vi "PWM_OUT.vi"() -> ()   [LabVIEW 2012]
uses:
  Usb_Daq_V52_Dll.dll
panel:
  in  "stop":bool
  in  "OK Button":bool
  in  "停止/运行":i32 min=0 max=1
  in  "占空比":sgl=1.0 min=1 max=99
  in  "频率":i32=1 min=1 max=100000
  in  "通道":i32=1 min=0 max=3
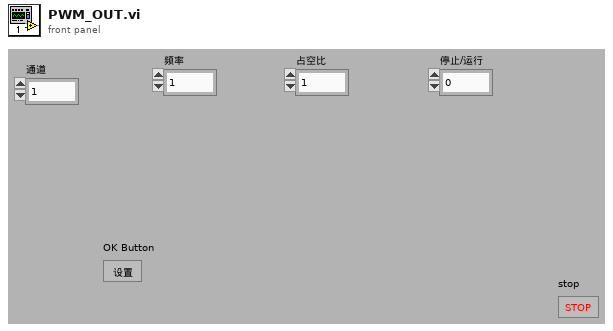
[diagram p1: front panel]
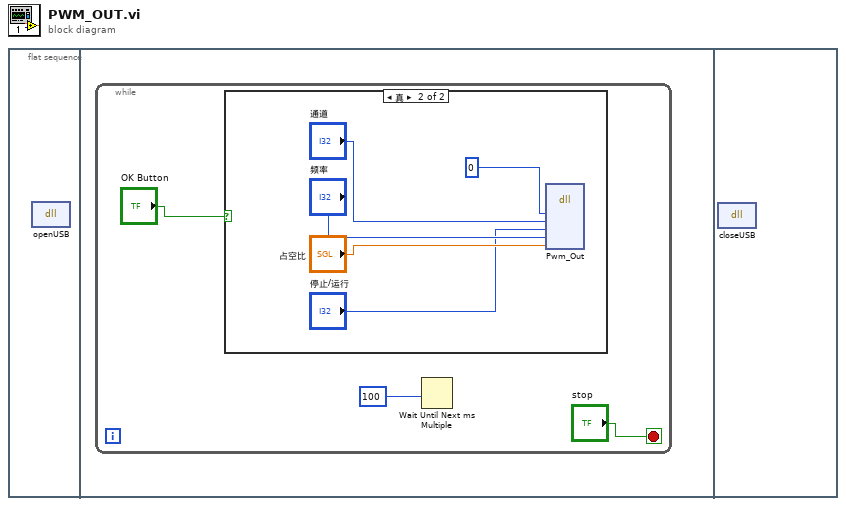
[diagram p0: block diagram]
diagram:
  n1 = flat-sequence {
    frame #0 {
      n2 = dll-call lib="PTH1labs Ebackup数据采集卡uSB!USB数据采集卡资料HKUSB6203例程labviewUsb_Daq_V52_Dll.dll" fn="openUSB"() -> ()  [unwired: 3 in, 3 out]
    }
    frame #1 {
      n3 = while {
        stop <- "stop" stop-if-true
        n4 = case shown="真" "OK Button" {
          frame False {
          }
          frame True {
            n5 = dll-call lib="PTH1labs Ebackup数据采集卡uSB!USB数据采集卡资料HKUSB6203例程labviewUsb_Daq_V52_Dll.dll" fn="Pwm_Out"("dev"=0, "chan"="通道", "en"="停止/运行", "freq"="频率", "DutyCycle"="占空比") -> ()  [unwired: 7 in, 4 out]
          }
        }
        n6 = Wait Until Next ms Multiple(millisecond multiple=100) -> ()  [unwired: 1 out]
      }
    }
    frame #2 {
      n7 = dll-call lib="PTH1labs Ebackup数据采集卡uSB!USB数据采集卡资料HKUSB6203例程labviewUsb_Daq_V52_Dll.dll" fn="closeUSB"() -> ()  [unwired: 3 in, 3 out]
    }
  }
